vi "Main - Get Local IP.vi"(8 "error in":errorcluster) -> (0 "error out":errorcluster)   [LabVIEW 2019]
uses:
  Controls/Global - Data UDP.vi
panel:
  out "standard output":string
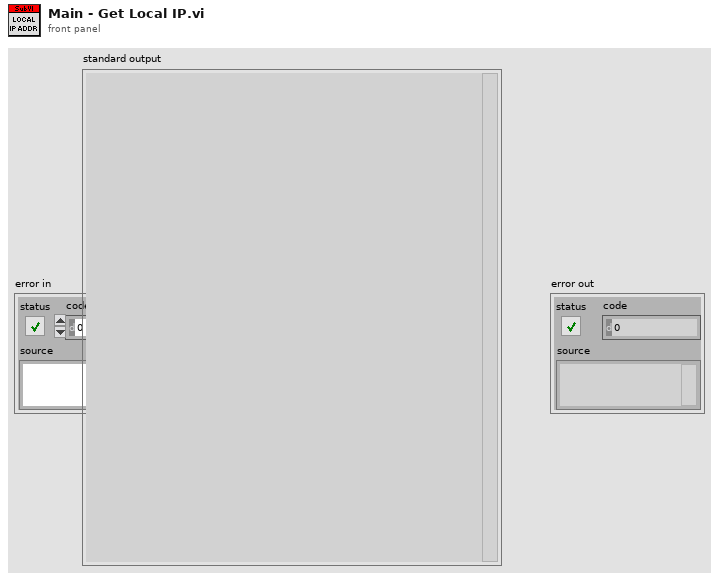
[diagram p1: front panel]
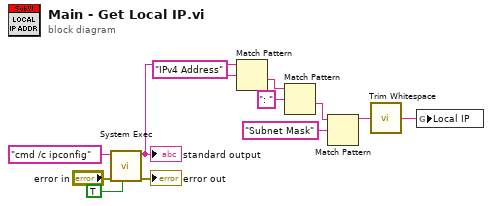
[diagram p0: block diagram]
diagram:
  n1 = call <vilib>:"System Exec.vi"("run minimized? (F)"=TRUE, "error in (no error)"="error in", "command line"="cmd /c ipconfig") -> ("error out"=→"error out":errorcluster, "standard output"=w8:string)  [unwired: 5 in, 2 out]
  "standard output" <- w8
  n2 = Match Pattern(string=w8, regular expression="IPv4 Address" ("search string")) -> (after substring=w6:string)  [unwired: 1 in, 3 out]
  n3 = Match Pattern(string=w6, regular expression=": ") -> (after substring=w3:string)  [unwired: 1 in, 3 out]
  n4 = Match Pattern(string=w3, regular expression="Subnet Mask") -> (before substring=w2:string)  [unwired: 1 in, 3 out]
  n5 = call <vilib>:"Trim Whitespace.vi"("string"=w2) -> ("trimmed string"=w1:string)  [unwired: 1 in]
  n6 = global write "Global - Data UDP.vi" "Local IP"(w1) -> ()
